vi "TEST_r_w_L1_oscar.vi"() -> ()   [LabVIEW 2012]
panel:
  out "error out":errorcluster
  out "data read value":u32=36
  in  "Data":i32
  in  "Register or channel":i32=96
  out "data out serial":string="0_2-63@36\r\n"
  in  "RD/#WR":bool
  in  "error in (no error)":errorcluster
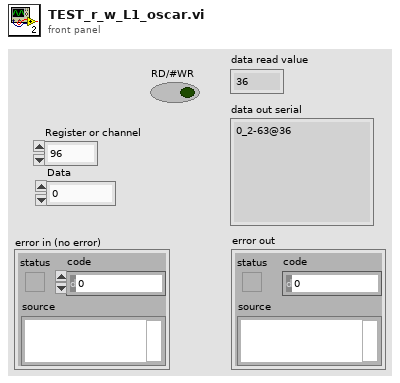
[diagram p1: front panel]
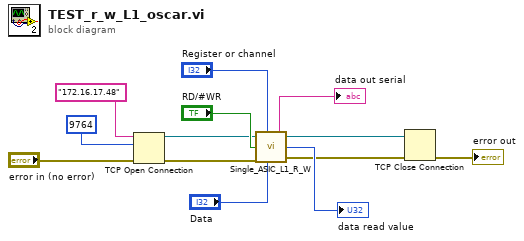
[diagram p0: block diagram]
diagram:
  n1 = TCP Open Connection(address="172.16.17.48", remote port or service name=9764, error in (no error)="error in (no error)") -> (connection ID=w1:refnum<k5>, error out=w2:errorcluster)  [unwired: 2 in]
  n2 = call "Single_ASIC_L1_R_W.vi"("connection ID"=w1, "Register or channel"="Register or channel", "RD/#WR"="RD/#WR", "error in (no error)"=w2, "Data"="Data") -> ("data out serial"=→"data out serial":string, "connection ID out"=w3:refnum<k5>, "data read value"=→"data read value":u32, "error out"=w4:errorcluster)  [unwired: 1 in]
  n3 = TCP Close Connection(connection ID=w3, error in (no error)=w4) -> (error out=→"error out":errorcluster)  [unwired: 1 in, 1 out]
